vi "CleanHandler.set clean time.vi"(0 "i ref in":refnum<vi>, 2 "clean time [s]":dbl format="%.2f", 3 "ms timeout (100)":i32=100, 5 "error in (no error)":errorcluster) -> (14 "i ref out":refnum<vi>, 17 "timed out":bool, 19 "error out":errorcluster)   [LabVIEW 2014, in "CleanHandler.lvlib"]
doc: "Sets the time used for cleaning. This time determines the length of the Gaussian waveform produced by one of the function generators."
uses:
  CleanHandler.lvlib
  CS_Core/CSSystem/CoreDefs/CoreDefs.error_type.ctl
  CS_Core/CSSystem/CoreLib/CoreLib.double 2 byte array.vi
  CS_Core/BaseProcess/BaseProcess.lvlib
  CS_Core/CSSystem/CoreLib/CoreLib.lvlib
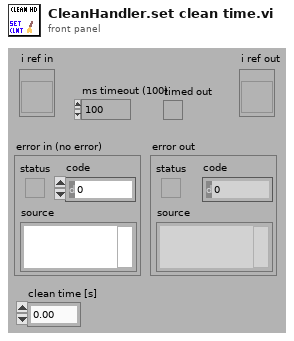
[diagram p1: front panel]
types:
  T1 = typedef "CoreDefs.error_type.ctl" = enum16{"no error", "can't load process", "can't unload process", "process does not exist", "can't install process", "can't remove process", "unknown function", "time out", "can't execute function", "duplicate queue name", "super not found", "caller queue invalid", "can't ping process", "unknown error", "VISA Error", "VISA timeout", "GPIB timeout", "GPIB error", "communication error", "data type mismatch", "can't read data from OPC server", "can't write data to OPC server", "OET error", "function not implemented", "process already exists", "invalid Shared Variable name", "error writing Shared Variable", "error reading Shared Variable", "invalid client name", "corrupt database", "unknown class", "call not authorized", "parameter out of range", "OET timeout: can't get data to modify", "invalid queue name", "requested operation incompatible with current state", "event undefined", "event disabled", "state undefined", "caller is not a friend", "EventBuilder: bad eventID", "EventBuilder: no DAQ devices", "a thread must not stop itself", "UNUSED ELEMENT4", "DiscArchiver: eventData incomplete", "DiscArchiver: eventData does not belong to run", "DiscArchiver: can't open file", "DiscArchiver: can't write to file", "DiscArchiver: available disc space low", "can't acquire semaphore", "error reading data from database", "notifier object is not existing", "can't register process", "can't unregister process", "illegal event type", "object disabled", "object already exists", "can't change state", "Instrument not found", "no connection to remote node", "invalid reference", "N/A", "UNUSED ELEMENT 1", "element not found", "illegal TCP/IP connection detected", "object does not exist", "invalid access ID", "unknown CS system", "invalid privilige", "unsupported data type", "unsupported server type", "IO server already exists", "Shared Variable already exists"}
  T2 = enum16{"simple", "synchronous", "asynchronous", "notification"}
  T3 = typedef "CoreDefs.rawDataType.ctl" = i8[]
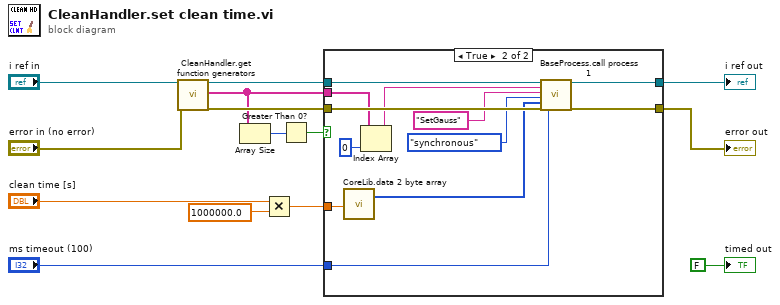
[diagram p0: block diagram]
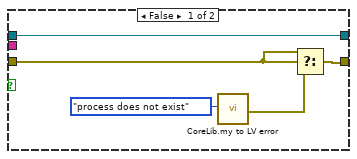
[diagram p2: hidden frame]
diagram:
  n1 = call "CleanHandler.get function generators.vi"("i ref in"="i ref in", "error in (no error)"="error in (no error)") -> ("i ref out"=w10:refnum<vi>, "function generators"=w5:string[], "error out"=w8:errorcluster)  [unwired: 14 in, 1 out]
  n2 = Array Size(array=w5) -> (size(s)=w12:i32)
  n3 = Multiply(x="clean time [s]", y=1000000.0) -> (x*y=w2:dbl)
  n4 = Greater Than 0?(x=w12) -> (x > 0?=w11:bool)
  n5 = case shown="True" w11 {
    tunnel: w10 -> [w15 w31]
    tunnel: "ms timeout (100)" -> [_ w30]
    tunnel: w8 -> [w18 w29]
    tunnel: [w19 w28] -> w7
    tunnel: [w15 w27] -> w6
    tunnel: w5 -> [_ w26]
    tunnel: w2 -> [_ w21]
    frame False {
      n6 = call "CoreLib.my to LV error.vi"("ErrorTypes"=CoreDefs.error_type."process does not exist") -> ("myErrorCluster"=w17:errorcluster)  [unwired: 17 in, 1 out]
      n7 = Select(t=w18, s=w18, f=w17) -> (s? t:f=w19:errorcluster)
    }
    frame True {
      n8 = call-poly "CoreLib.data 2 byte array.vi"("f64"=w21) -> ("byteArray out"=w20:T3)  [unwired: 18 in]
      n9 = Index Array(array=w26, index=0) -> (element=w25:string)
      n10 = call "BaseProcess.call process 1.vi"("i ref in"=w31, "Object"=w25, "Selector"="SetGauss", "CallType"=T2."synchronous", "Data"=w20, "error in (no error)"=w29, "timeout (ms)"=w30) -> ("i ref out"=w27:refnum<vi>, "error out"=w28:errorcluster)  [unwired: 10 in, 1 out]
    }
  }
  "error out" <- w7
  "i ref out" <- w6
  "timed out" <- FALSE ("timed out")
